vi "print scan sheet labels.vi"() -> ()   [LabVIEW 2013]
panel:
  out "error out":errorcluster
  in  "Printer name":string="\\\\dt-hkn77p2\\ZDesigner ZT230-200dpi ZPL"
  out "text lines":string[](array[string])
  in  "error in":errorcluster
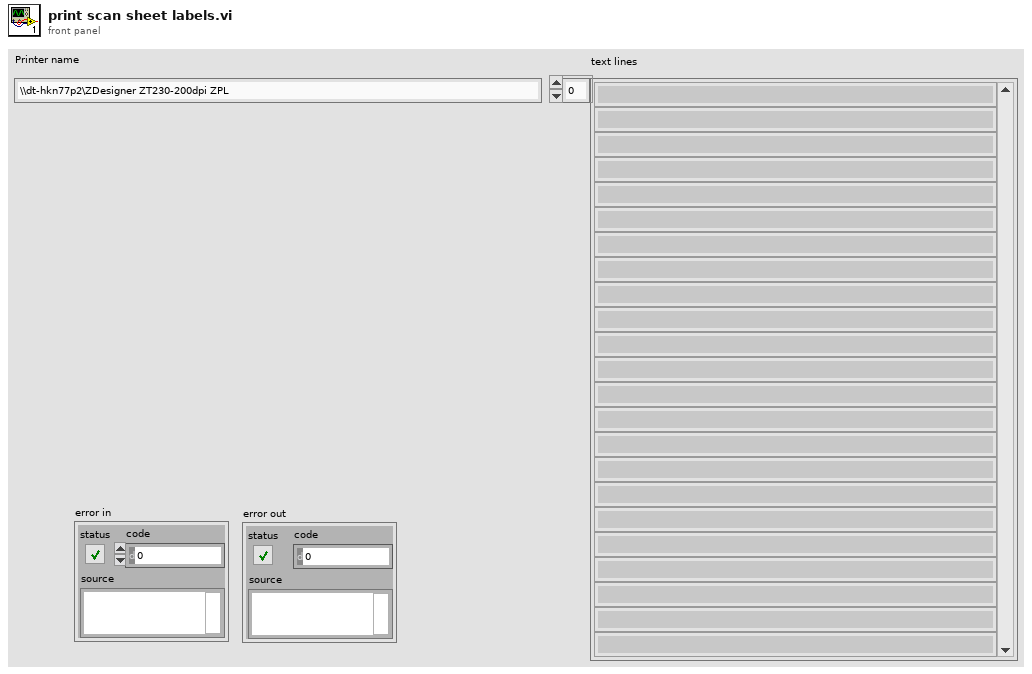
[diagram p1: front panel]
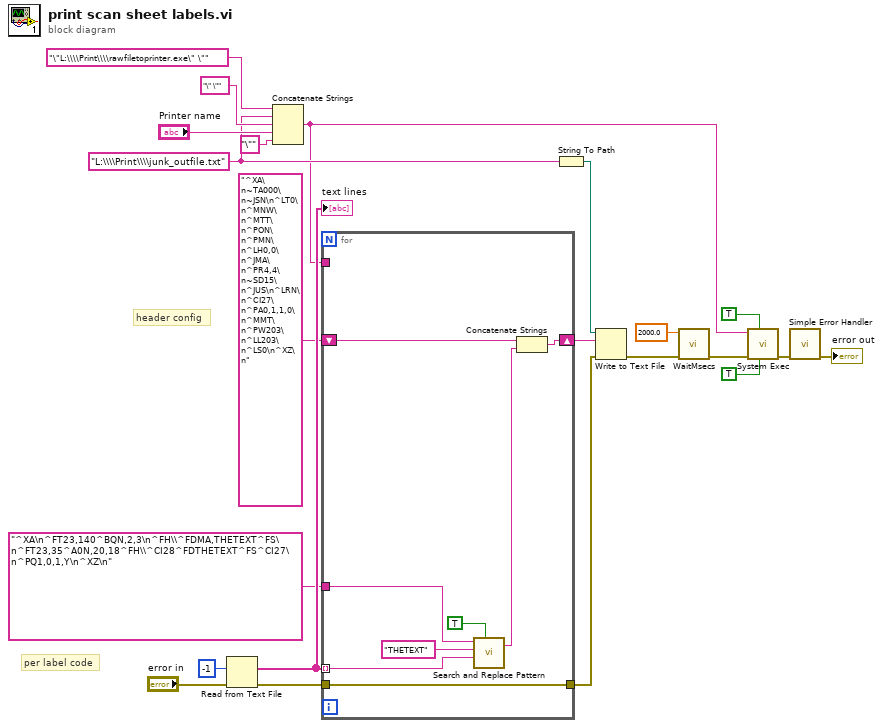
[diagram p0: block diagram]
diagram:
  w4 = "L:\\\\Print\\\\junk_outfile.txt" ("string")
  # "per label code"
  # "header config"
  n1 = Read from Text File(count=-1, error in="error in") -> (text=w20:string[], error out=w19:errorcluster)  [unwired: 2 in, 2 out]
  "text lines" <- w20
  n2 = Concatenate Strings("\"L:\\\\Print\\\\rawfiletoprinter.exe\" \"" ("string"), w4, "\" \"" ("string"), "Printer name", "\"" ("string")) -> (w2:string)
  n3 = for {
    tunnel: w20 -> [w29] mode=indexing
    tunnel: w19 -> [w23]
    tunnel: w2 -> [_]
    shift-right: [w24] -> w5
    shift-left: "^XA\n~TA000\n~JSN\n^LT0\n^MNW\n^MTT\n^PON\n^PMN\n^LH0,0\n^JMA\n^PR4,4\n~SD15\n^JUS\n^LRN\n^CI27\n^PA0,1,1,0\n^MMT\n^PW203\n^LL203\n^LS0\n^XZ\n" -> [w26]
    tunnel: "^XA\n^FT23,140^BQN,2,3\n^FH\\^FDMA,THETEXT^FS\n^FT23,35^A0N,20,18^FH\\^CI28^FDTHETEXT^FS^CI27\n^PQ1,0,1,Y\n^XZ\n" -> [w27]
    tunnel: [w23] -> w7
    n4 = call <vilib>:"Search and Replace Pattern.vi"("string"=w27, "regular expression (\"\")"="THETEXT" ("regular expression (\"\")"), "replace string (\"\")"=w29, "replace all? (F)"=TRUE) -> ("result string"=w25:string)  [unwired: 1 in, 1 out]
    n5 = Concatenate Strings(w26, w25) -> (w24:string)
  }
  n6 = String To Path(string=w4) -> (path=w3:path)
  n7 = Write to Text File(file (use dialog)=w3, text=w5, error in=w7) -> (error out=w14:errorcluster)  [unwired: 1 in, 2 out]
  n8 = call "WaitMsecs.vi"("error in (no error)"=w14, "Wait Msecs"=2000.0) -> ("error out"=w12:errorcluster)  [unwired: 9 in]
  n9 = call <vilib>:"System Exec.vi"("run minimized? (F)"=TRUE, "wait until completion? (T)"=TRUE, "error in (no error)"=w12, "command line"=w2) -> ("error out"=w11:errorcluster)  [unwired: 4 in, 3 out]
  n10 = call <vilib>:"Simple Error Handler.vi"("error in (no error)"=w11) -> ("error out"=→"error out":errorcluster)  [unwired: 4 in, 4 out]
